vi "testing.vi"() -> ()   [LabVIEW 2019]
uses:
  <vilib>/imath/engines/lvmath2/RunTimeEngine/Managers/WorkSpace/UID Generator.vi
  <vilib>/imath/engines/lvmath2/RunTimeEngine/RunTimeType/NIMS_RunTimeType_From StrictType (excl LVString).vi
  <instcachedir>/0/NIMS_RunTimeType_From StrictType (excl LVString)_6DA94F09978249AAA8963F8D3C6FF051.lvgen/NIMS_RunTimeType_From StrictType (excl LVString)_6DA94F09978249AAA8963F8D3C6FF051_000.vi
  <vilib>/imath/engines/lvmath2/RunTimeEngine/LocalVariableDefStatement/MC_LocalVariableDefStatement_Display.vi
  <vilib>/imath/engines/lvmath2/RunTimeEngine/Managers/SymbolTable/Clear UID.vi
  <vilib>/imath/engines/lvmath2/RunTimeEngine/NodeEndStatement/NIMS_NodeEndStatement_Output.vi
  <instcachedir>/0/NIMS_NodeEndStatement_Output_53EC0D466D134D7ABD903AC30B43404B.lvgen/NIMS_NodeEndStatement_Output_53EC0D466D134D7ABD903AC30B43404B_001.vi
  <vilib>/imath/engines/lvmath2/RunTimeEngine/ErrorHandling/NIMS_Finalize Error.vi
  <vilib>/imath/engines/lvmath2/RunTimeEngine/Managers/SymbolTable/NIMS_WorkSpace.lvlib
panel:
  in  "ON/OFF":bool
  out "General Alarm":bool
  out "Smoke Alarm":bool
  out "Temperature Alarm":bool
  in  "Smoke Level Detector":dbl(slide) scale=0.0..1000.0
  in  "Thermometer":dbl(slide) scale=0.0..1000.0
  out "Richter Scale Meter":dbl(knob) scale=0.0..10.0
  out "Earthquake":bool
  out "Tsunami":bool
  out "Normal":bool
  out "x+y":i32
  out "M (Richter Scale)":dbl
  in  "Amplitude (1*10^-6 m)":dbl
  in  "Distance (1*10^3 m)":dbl
  # "Fire Alarm"
  # "Earth Quake and Tsunami Alarm"
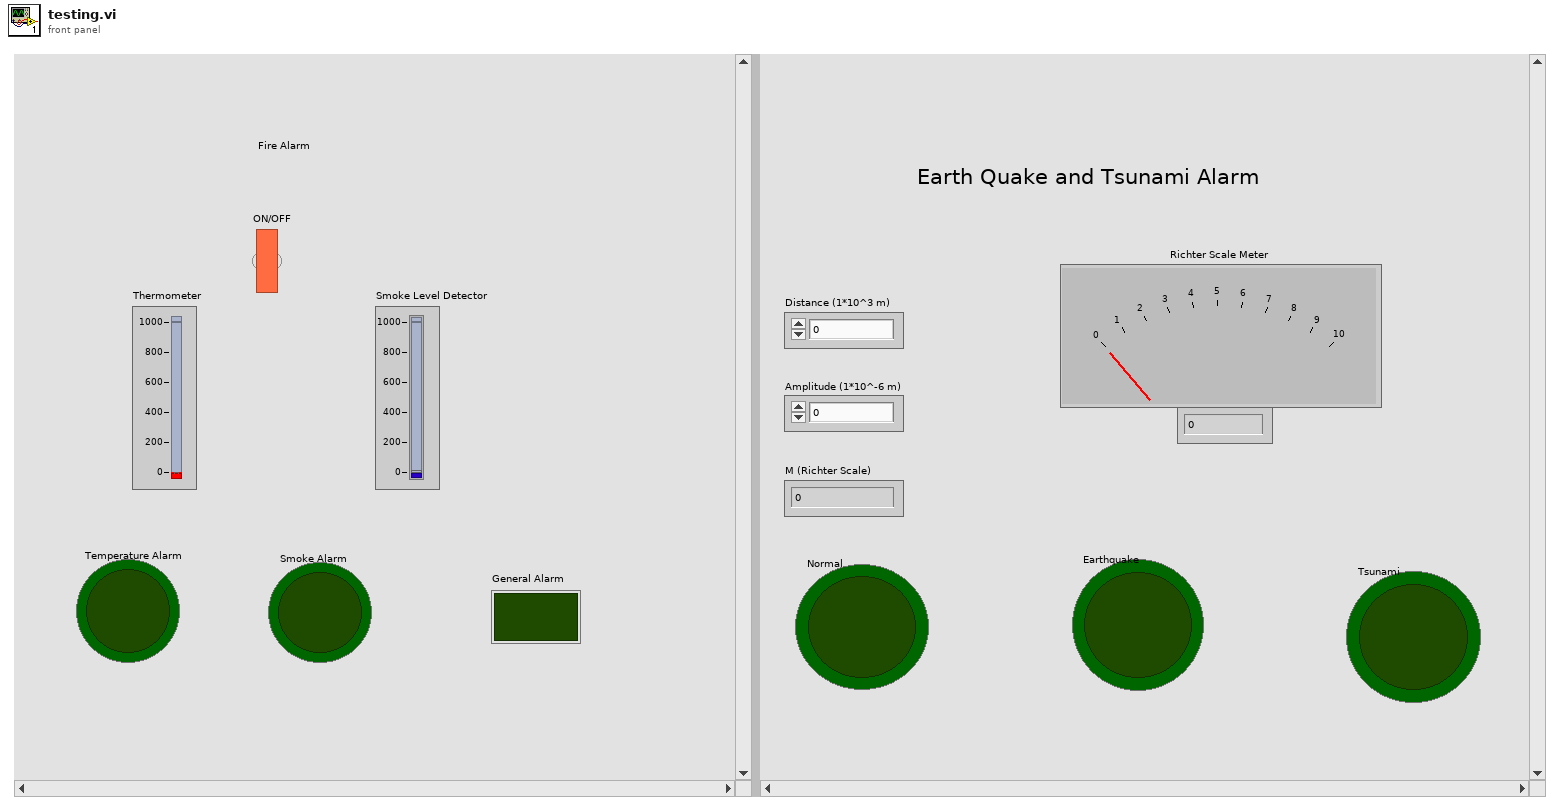
[diagram p1: front panel]
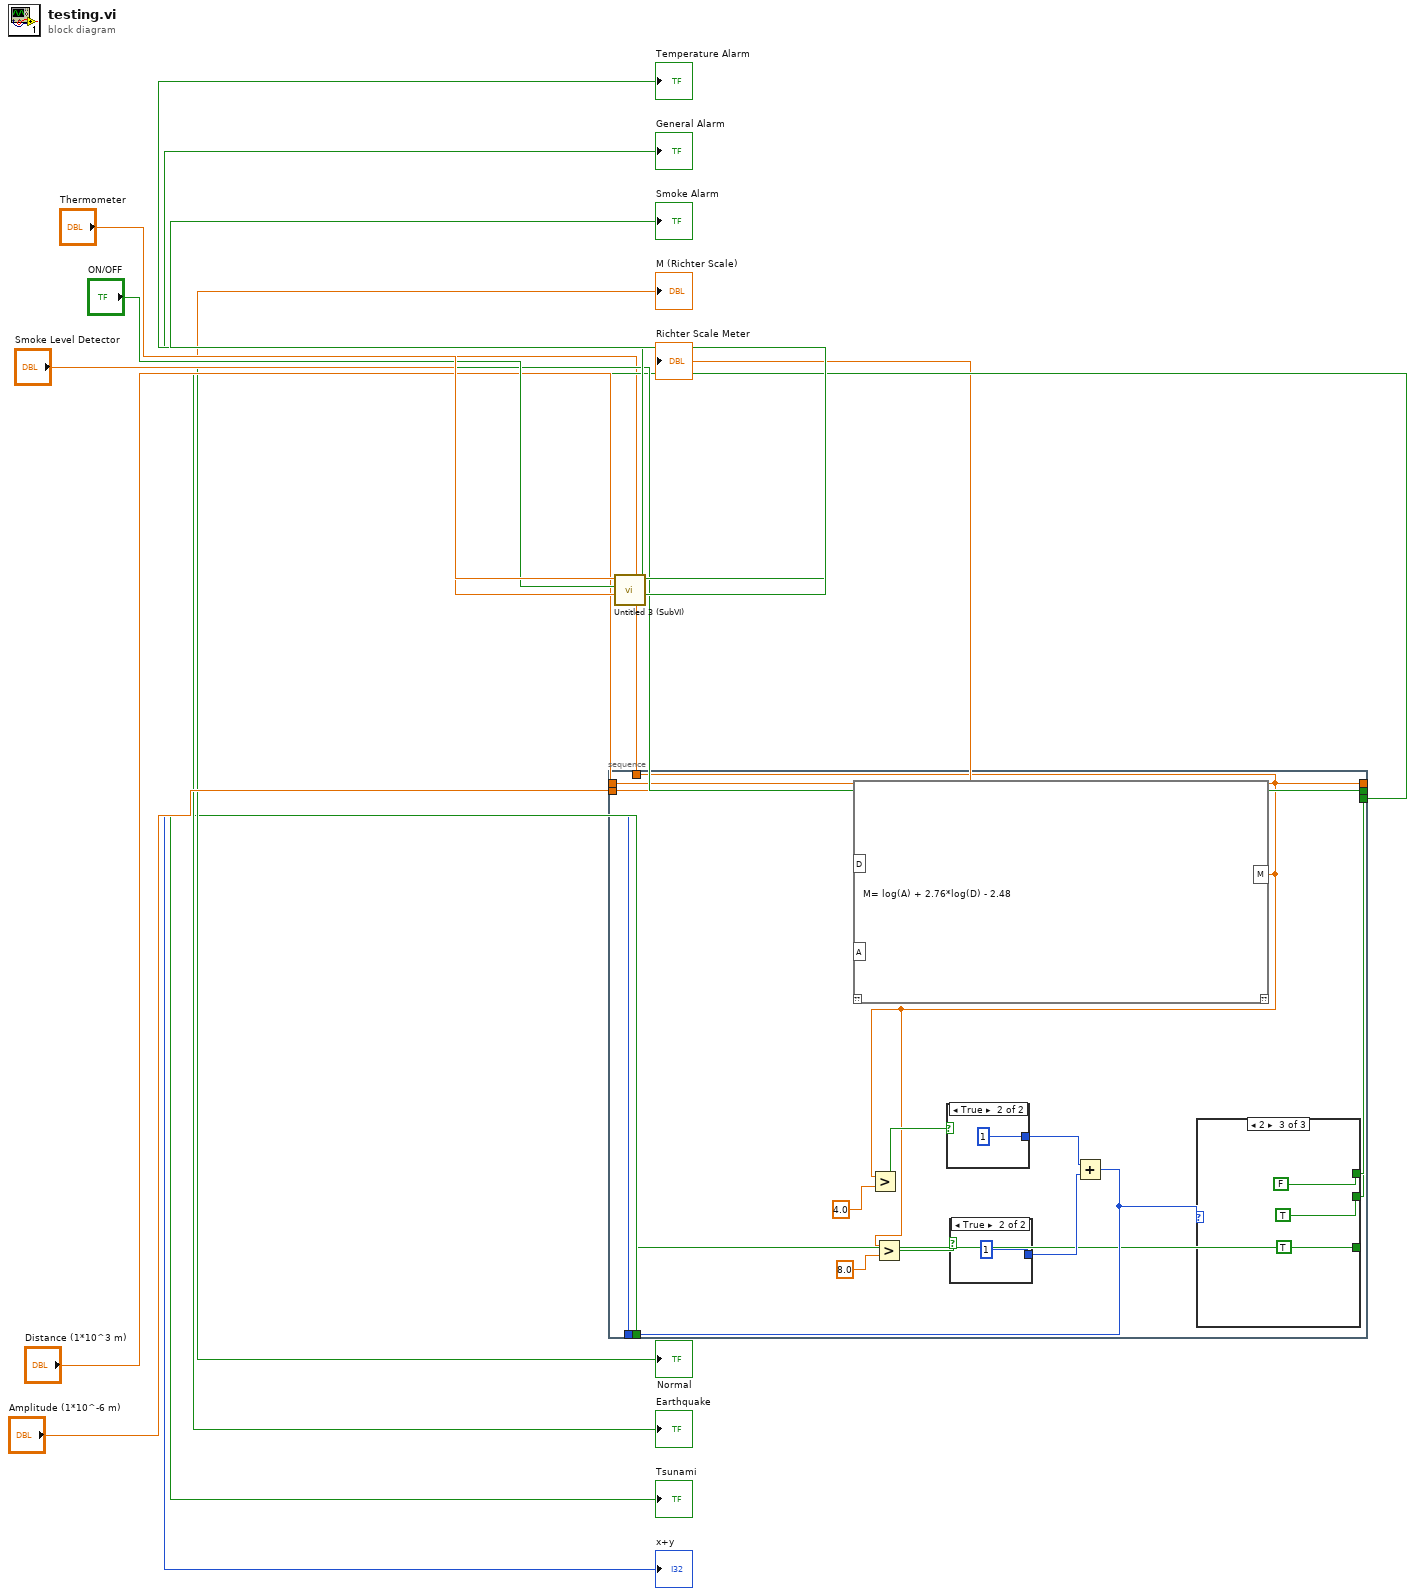
[diagram p0: block diagram]
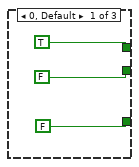
[diagram p2: hidden frame]
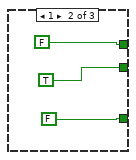
[diagram p3: hidden frame]
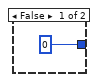
[diagram p4: hidden frame]
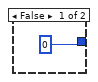
[diagram p5: hidden frame]
diagram:
  n1 = stacked-sequence {
    tunnel: [w17] -> w5
    tunnel: [w18] -> w6
    tunnel: [w15] -> w2
    tunnel: [w16] -> w4
    tunnel: [w15] -> w3
    tunnel: [w19] -> w1
    tunnel: "Amplitude (1*10^-6 m)" -> [w26]
    tunnel: "Distance (1*10^3 m)" -> [w27]
    frame #0 {
      n2 = mathscript code="M= log(A) + 2.76*log(D) - 2.48"("D"=w27, "A"=w26) -> ("M"=w15:dbl)  [unwired: 1 in, 1 out]
      n3 = Greater?(x=w15, y=4.0) -> (0:w23:bool)
      n4 = Greater?(x=w15, y=8.0) -> (0:w22:bool)
      n5 = case shown="True" w23 {
        tunnel: [0 1] -> w21
        frame False {
        }
        frame True {
        }
      }
      n6 = case shown="True" w22 {
        tunnel: [0 1] -> w20
        frame False {
        }
        frame True {
        }
      }
      n7 = Add(x=w21, y=w20) -> (x+y=w19:i32)
      n8 = case shown="2" w19 {
        tunnel: [TRUE FALSE FALSE] -> w18
        tunnel: [FALSE TRUE TRUE] -> w17
        tunnel: [FALSE FALSE TRUE] -> w16
        frame 0, Default {
        }
        frame 1 {
        }
        frame 2 {
        }
      }
    }
  }
  "M (Richter Scale)" <- w3
  "x+y" <- w1
  "Normal" <- w6
  "Tsunami" <- w4
  "Earthquake" <- w5
  "Richter Scale Meter" <- w2
  n9 = call "Untitled 3 (SubVI).vi"("Smoke Level Detector"="Smoke Level Detector", "ON/OFF"="ON/OFF", "Thermometer"="Thermometer") -> ("Boolean 3"=→"Smoke Alarm":bool, "Boolean"=→"General Alarm":bool, "Boolean 2"=→"Temperature Alarm":bool)  [unwired: 6 in]
